vi "newfiles.vi"   [LabVIEW 2022 SP3]
types:
  T1 = enum16{"open", "replace", "create", "open or create", "replace or create", "replace or create with confirmation"}
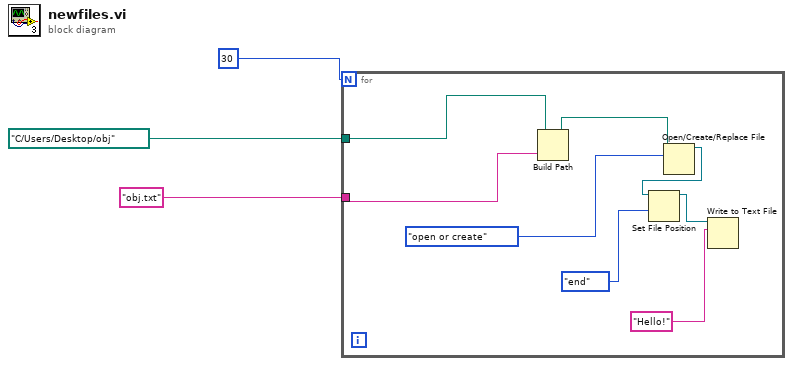
[diagram p0: block diagram]
diagram:
  n1 = for {
    N: 30 -> [_]
    tunnel: path "C:/Users/Desktop/obj" -> [w11]
    tunnel: "obj.txt" -> [w10]
    n2 = Build Path(base path=w11, name or relative path=w10) -> (appended path=w8:path)
    n3 = Open/Create/Replace File(file path (use dialog)=w8, operation (0:open)=T1."open or create" ("操作(0:open)")) -> (refnum out=w7:refnum<file>)  [unwired: 4 in, 2 out]
    n4 = Set File Position(refnum=w7, from (0:start)=enum16{"start", "end", "current"}."end" ("自（0:起始）")) -> (refnum out=w6:refnum<file>)  [unwired: 2 in, 1 out]
    n5 = Write to Text File(file (use dialog)=w6, text="Hello!") -> ()  [unwired: 2 in, 3 out]
  }
